vi "FT10_M4X Configure Vertical.vi"(0 "Card Handle in":u32, 5 "Channel":enum16{"CH0", "CH1", "CH2", "CH3"}(ring), 7 "Range":T1(ring), 9 "Offset (% of Range)":i32, 11 "error in (no error)":errorcluster) -> (4 "Card Handle out":u32, 15 "error out":errorcluster)   [LabVIEW 2024]
doc: "Copy of \"M4X_Configure Vertical.vi\" from HWT_Lillis_7854.lvproj"
uses:
  LV2015/Transfer dlls/spcm_win32.dll
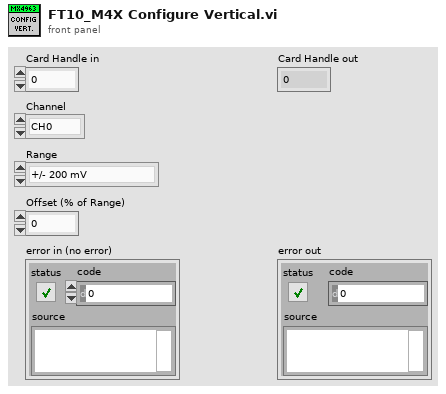
[diagram p1: front panel]
types:
  T1 = enum16{"+/- 200 mV", "+/- 500 mV", "+/- 1 V", "+/- 2 V", "+/- 5 V", "+/- 10 V"}
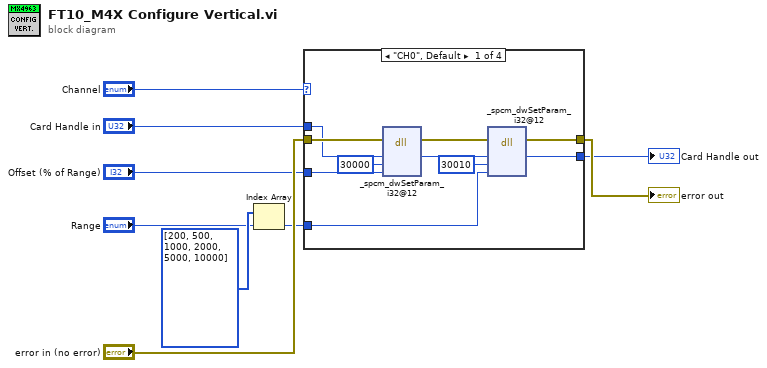
[diagram p0: block diagram]
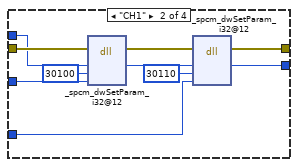
[diagram p2: hidden frame]
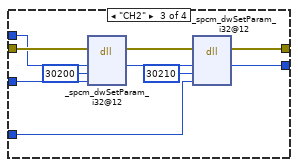
[diagram p3: hidden frame]
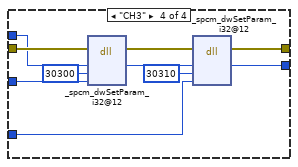
[diagram p4: hidden frame]
diagram:
  n1 = Index Array(array=i32[] [200, 500, 1000, 2000, 5000, 10000], index="Range") -> (element=w5:i32)
  n2 = case shown="\"CH0\", Default" "Channel" {
    tunnel: "Offset (% of Range)" -> [w16 w26 w36 w46]
    tunnel: "Card Handle in" -> [w18 w28 w38 w48]
    tunnel: w5 -> [w13 w23 w33 w43]
    tunnel: "error in (no error)" -> [w19 w29 w39 w49]
    tunnel: [w11 w21 w31 w41] -> w9
    tunnel: [w10 w20 w30 w40] -> w8
    frame "CH0", Default {
      n3 = dll-call lib="C:/Users/yearon2/OneDrive - Medtronic PLC/LV2015/Transfer dlls/spcm_win32.dll" fn="_spcm_dwSetParam_i32@12" label="Set Offset"(error in=w19, "hDrv"=w18, "lRegister"=30000 ("Reg"), "lValue"=w16) -> (error out=w12:errorcluster, "hDrv"=w14:u32)  [unwired: 5 in, 1 out]
      n4 = dll-call lib="C:/Users/yearon2/OneDrive - Medtronic PLC/LV2015/Transfer dlls/spcm_win32.dll" fn="_spcm_dwSetParam_i32@12" label="Set Input Range"(error in=w12, "hDrv"=w14, "lRegister"=30010 ("Reg"), "lValue"=w13) -> (error out=w11:errorcluster, "hDrv"=w10:u32)  [unwired: 5 in, 1 out]
    }
    frame "CH1" {
      n5 = dll-call lib="C:/Users/yearon2/OneDrive - Medtronic PLC/LV2015/Transfer dlls/spcm_win32.dll" fn="_spcm_dwSetParam_i32@12" label="Set Offset"(error in=w29, "hDrv"=w28, "lRegister"=30100 ("Reg"), "lValue"=w26) -> (error out=w22:errorcluster, "hDrv"=w24:u32)  [unwired: 5 in, 1 out]
      n6 = dll-call lib="C:/Users/yearon2/OneDrive - Medtronic PLC/LV2015/Transfer dlls/spcm_win32.dll" fn="_spcm_dwSetParam_i32@12" label="Set Input Range"(error in=w22, "hDrv"=w24, "lRegister"=30110 ("Reg"), "lValue"=w23) -> (error out=w21:errorcluster, "hDrv"=w20:u32)  [unwired: 5 in, 1 out]
    }
    frame "CH2" {
      n7 = dll-call lib="C:/Users/yearon2/OneDrive - Medtronic PLC/LV2015/Transfer dlls/spcm_win32.dll" fn="_spcm_dwSetParam_i32@12" label="Set Offset"(error in=w39, "hDrv"=w38, "lRegister"=30200 ("Reg"), "lValue"=w36) -> (error out=w32:errorcluster, "hDrv"=w34:u32)  [unwired: 5 in, 1 out]
      n8 = dll-call lib="C:/Users/yearon2/OneDrive - Medtronic PLC/LV2015/Transfer dlls/spcm_win32.dll" fn="_spcm_dwSetParam_i32@12" label="Set Input Range"(error in=w32, "hDrv"=w34, "lRegister"=30210 ("Reg"), "lValue"=w33) -> (error out=w31:errorcluster, "hDrv"=w30:u32)  [unwired: 5 in, 1 out]
    }
    frame "CH3" {
      n9 = dll-call lib="C:/Users/yearon2/OneDrive - Medtronic PLC/LV2015/Transfer dlls/spcm_win32.dll" fn="_spcm_dwSetParam_i32@12" label="Set Offset"(error in=w49, "hDrv"=w48, "lRegister"=30300 ("Reg"), "lValue"=w46) -> (error out=w42:errorcluster, "hDrv"=w44:u32)  [unwired: 5 in, 1 out]
      n10 = dll-call lib="C:/Users/yearon2/OneDrive - Medtronic PLC/LV2015/Transfer dlls/spcm_win32.dll" fn="_spcm_dwSetParam_i32@12" label="Set Input Range"(error in=w42, "hDrv"=w44, "lRegister"=30310 ("Reg"), "lValue"=w43) -> (error out=w41:errorcluster, "hDrv"=w40:u32)  [unwired: 5 in, 1 out]
    }
  }
  "Card Handle out" <- w8
  "error out" <- w9
